vi "myRIO_BRig_FPGA_v3,80__PortC.vi"() -> ()   [LabVIEW 2014]
uses:
  <vilib>/rvi/Emulation/niFpgaGetClockAttributes.vi
  <vilib>/rvi/Emulation/niFpgaSctlEmulationGetInTimedLoop.vi
  <vilib>/rvi/Emulation/niFpgaEmulationReportErrorSimple.vi
  <vilib>/rvi/eio/common/nirviEmuTemplateMethod_errors.vi
  <vilib>/rvi/Emulation/niFpgaCriticalErrorInLSC.vi
  <vilib>/eio/EIONode/EIONode.xnode
panel:
  in  "I_allReward":bool
  in  "AnaOut_1":i16
  in  "CueLed_Event":bool
  in  "CueLed_nValley":u32=100
  in  "CueLed_nPeak":u32=100
  in  "LC_Event_l2":bool
  in  "LC_Laser_l2":bool
  in  "LC_nShutter_l2":u32=100
  in  "LC_nValley_l2":u32=100
  in  "LC_nPeak_l2":u32=100
  in  "LR_wrong_nDelay_l2":u32
  in  "LR_reward_nDelay_l2":u32
  in  "LR_wrong_nTotal_l2":u32=100
  in  "LR_reward_nTotal_l2":u32=100
  in  "LR_wrong_laser_l2":bool
  in  "LR_wrong_Event_l2":bool
  in  "LR_reward_Laser_l2":bool
  in  "LR_reward_Event_l2":bool
  out "AnaIn_1":i16
  out "AnaIn_0":i16
  out "timeTrial_count":u32
  in  "timeTrial_trig":bool
  in  "k1__counter_per_ms":u16=100 min=100 max=40000 step=1
  in  "LC_nShutter_l1":u32=100
  in  "AnaOut_0":i16
  in  "LC_nValley_l1":u32=100
  in  "LC_nPeak_l1":u32=100
  in  "LC_Event_l1":bool
  in  "LR_wrong_nTotal_l1":u32=100
  in  "LR_wrong_nDelay_l1":u32
  in  "LR_reward_nTotal_l1":u32=100
  in  "LR_reward_nDelay_l1":u32
  in  "LR_reward_Event_l1":bool
  in  "LR_wrong_Event_l1":bool
  out "SelectWrong":bool
  out "SelectReward":bool
  in  "LR_wrong_Laser_l1":bool
  in  "LR_reward_Laser_l1":bool
  in  "Left(F)_or_Right(T)":bool
  in  "ignoreWrong":bool
  in  "SelectionState":bool
  in  "LC_Laser_l1":bool
  in  "FPGA_Stop":bool
  in  "audioTrigger_L":bool
  in  "audioTrigger_R":bool
  in  "audioFreq_L_kHz":u8=14 min=1 max=14 step=1
  in  "audioAmp_L":u16=1 min=1 max=32767 step=1
  in  "audioFreq_R_kHz":u8=14 min=1 max=14 step=1
  in  "audioAmp_R":u16=1 min=1 max=32767 step=1
  in  "A3_SL":bool
  in  "A1_SR":bool
  in  "Counts_Reset":bool
  out "A4_LickR":u32
  out "A2_LickL":u32
  in  "A6_Act":bool
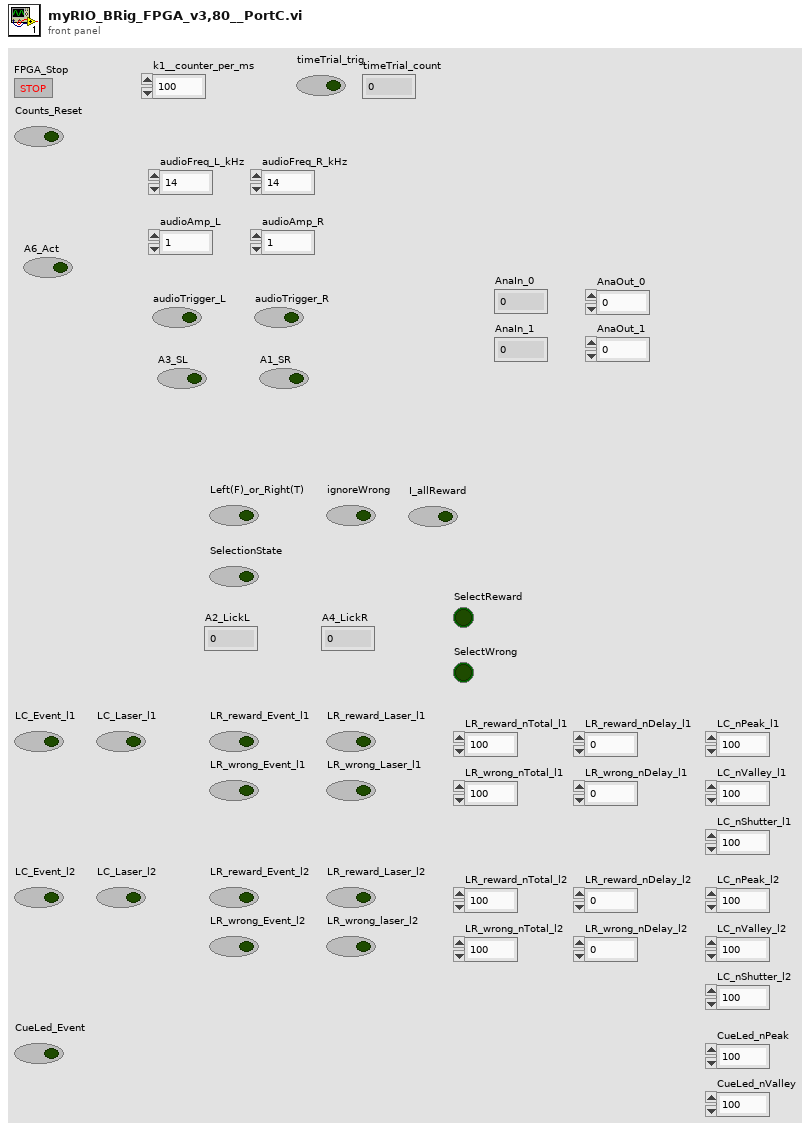
[diagram p1: front panel]
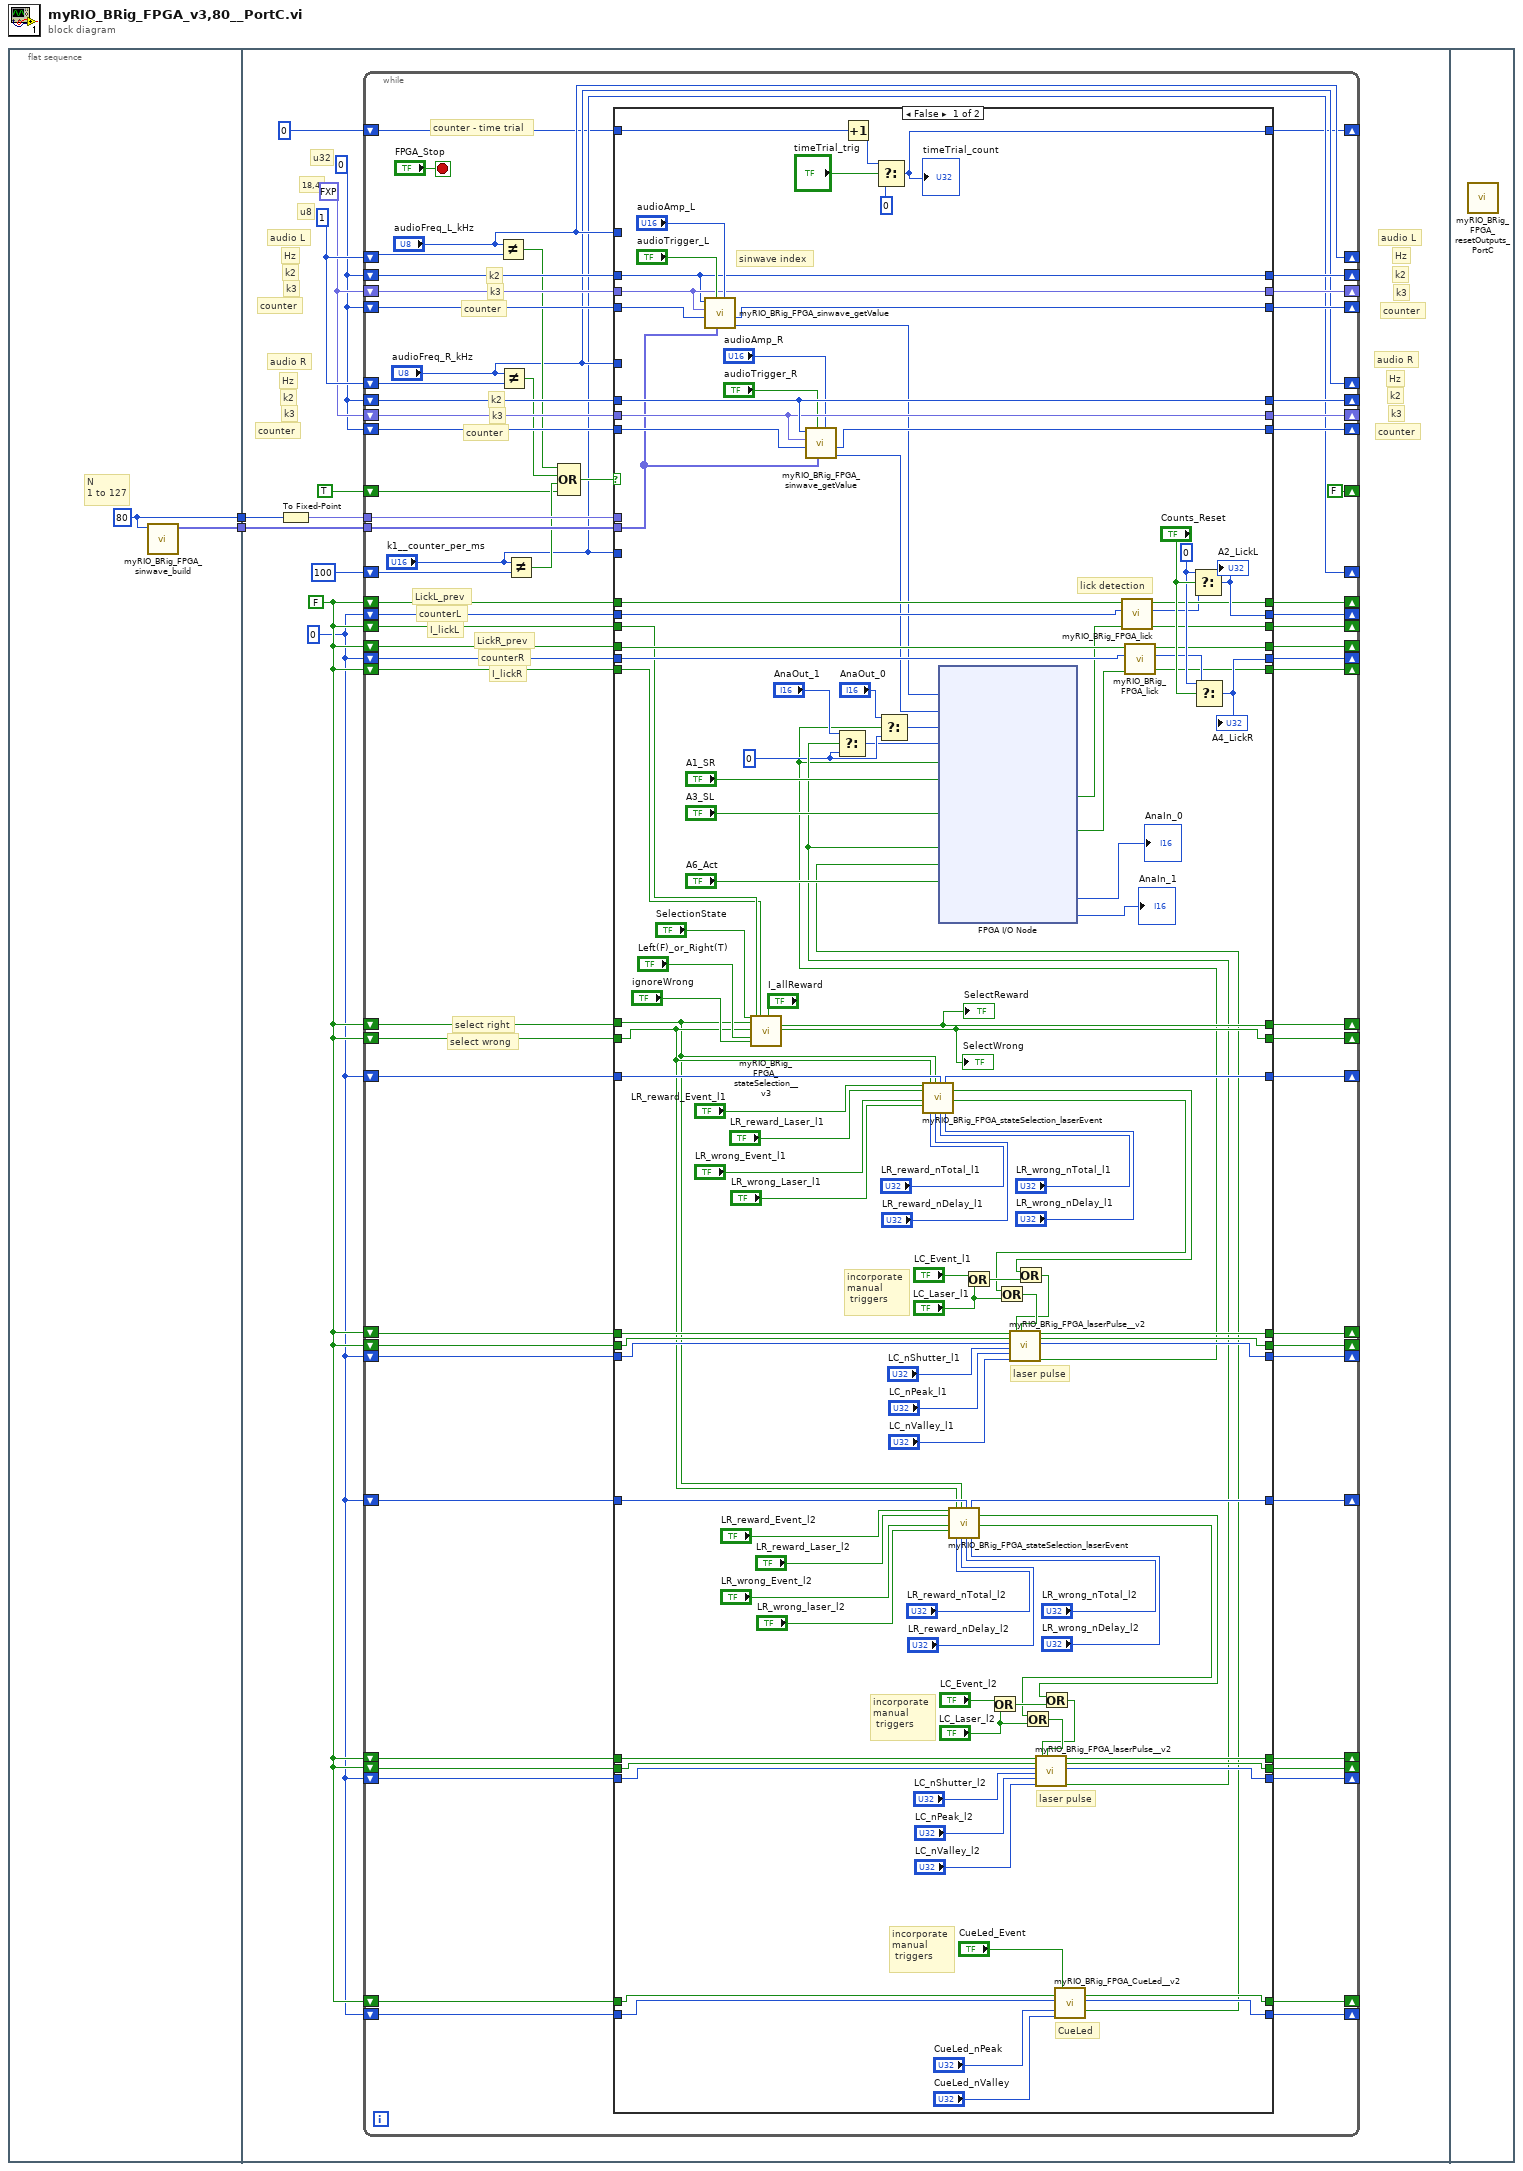
[diagram p0: block diagram]
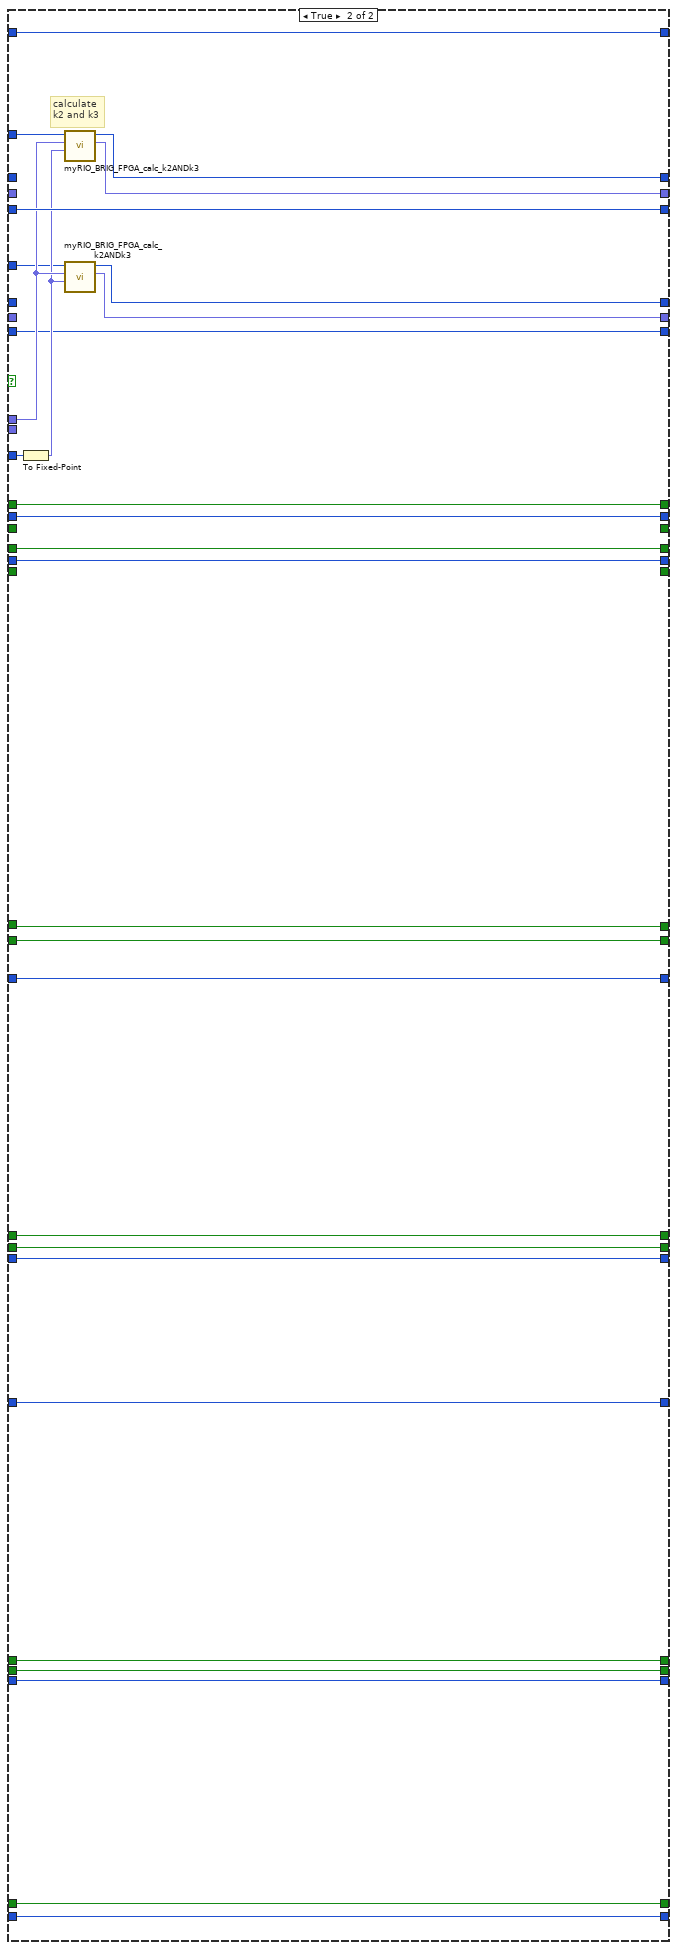
[diagram p2: hidden frame]
diagram:
  n1 = flat-sequence {
    tunnel: [w4] -> w2
    tunnel: [w3] -> w1
    tunnel: w2 -> [w15]
    tunnel: w1 -> [w14]
    frame #0 {
      w3 = 80 ("dimension size")
      # "N\n1 to 127"
      n2 = call "myRIO_BRig_FPGA_sinwave_build.vi"("input_Npts"=w3) -> ("output_array_sin"=w4:fxp<+/-,16,2>[])  [unwired: 10 in]
    }
    frame #1 {
      w5 = u32 0
      w6 = FALSE
      w10 = u32 0
      w11 = fxp<+,18,4> 0.0
      w12 = u8 1
      # "counter"
      # "k3"
      # "k2"
      # "counter"
      # "k3"
      # "k2"
      # "counter"
      # "counter"
      # "u32"
      # "k3"
      # "k2"
      # "k3"
      # "18,4"
      # "u8"
      # "Hz"
      # "Hz"
      # "audio R"
      # "audio L"
      # "Hz"
      # "k2"
      # "Hz"
      # "audio R"
      # "audio L"
      n3 = To Fixed-Point(number=w14) -> (fixed-point=w13:fxp<+,7,7>)  [unwired: 1 in]
      n4 = while {
        shift-right: ["audioFreq_L_kHz"] -> _
        shift-left: w12 -> [w80]
        shift-right: [w74] -> _
        shift-left: w10 -> [w78]
        shift-right: ["audioFreq_R_kHz"] -> _
        shift-left: w12 -> [w70]
        tunnel: w15 -> [w77]
        tunnel: w13 -> [w76]
        shift-right: [w73] -> _
        shift-left: w11 -> [w75]
        shift-right: [w71] -> _
        shift-left: w10 -> [w72]
        shift-right: [w68] -> _
        shift-left: w10 -> [w69]
        shift-right: [w66] -> _
        shift-left: w11 -> [w67]
        shift-right: [w64] -> _
        shift-left: w10 -> [w65]
        shift-right: ["k1__counter_per_ms"] -> _
        shift-left: u16 100 ("y") -> [w63]
        shift-right: [FALSE] -> _
        shift-left: TRUE -> [w58]
        shift-right: [w51] -> _
        shift-left: w6 -> [w53]
        shift-right: [w50] -> _
        shift-left: w6 -> [w52]
        shift-right: [w48] -> _
        shift-left: w5 -> [w49]
        shift-right: [w46] -> _
        shift-left: w5 -> [w47]
        shift-right: [w43] -> _
        shift-left: w6 -> [w45]
        shift-right: [w42] -> _
        shift-left: w6 -> [w44]
        shift-right: [w40] -> _
        shift-left: w6 -> [w41]
        shift-right: [w38] -> _
        shift-left: w6 -> [w39]
        shift-right: [w36] -> _
        shift-left: u32 0 -> [w37]
        shift-right: [w34] -> _
        shift-left: w5 -> [w35]
        shift-right: [w33] -> _
        shift-left: w6 -> [w30]
        shift-right: [w32] -> _
        shift-left: w6 -> [w29]
        shift-right: [w31] -> _
        shift-left: w5 -> [w28]
        shift-right: [w26] -> _
        shift-left: w5 -> [w27]
        shift-right: [w25] -> _
        shift-left: w6 -> [w22]
        shift-right: [w24] -> _
        shift-left: w6 -> [w21]
        shift-right: [w23] -> _
        shift-left: w5 -> [w20]
        shift-right: [w19] -> _
        shift-left: w6 -> [w17]
        shift-right: [w18] -> _
        shift-left: w5 -> [w16]
        stop <- "FPGA_Stop" stop-if-true
        # "counter"
        # "k3"
        # "k2"
        # "counter"
        # "k3"
        # "k2"
        # "counter - time trial"
        # "I_lickR"
        # "counterR"
        # "LickR_prev"
        # "I_lickL"
        # "counterL"
        # "LickL_prev"
        # "select wrong"
        # "select right"
        n5 = Not Equal?(x="audioFreq_L_kHz", y=w80) -> (x != y?=w62:bool)
        n6 = Not Equal?(x="audioFreq_R_kHz", y=w70) -> (x != y?=w61:bool)
        n7 = Not Equal?(x="k1__counter_per_ms", y=w63) -> (x != y?=w59:bool)
        n8 = Compound Arithmetic op=OR(w62, w61, w59, w58) -> (w60:bool)
        n9 = case shown="False" w60 {
          tunnel: w78 -> [w183 _]
          tunnel: "audioFreq_L_kHz" -> [_ w225]
          tunnel: w77 -> [w176 _]
          tunnel: w76 -> [_ w221]
          tunnel: "k1__counter_per_ms" -> [_ w226]
          tunnel: w75 -> [w184 _]
          tunnel: [w183 w224] -> w74
          tunnel: [w184 w223] -> w73
          tunnel: w72 -> [w188 w222]
          tunnel: [w185 w222] -> w71
          tunnel: w69 -> [w180 _]
          tunnel: [w180 w217] -> w68
          tunnel: w67 -> [w179 _]
          tunnel: [w179 w218] -> w66
          tunnel: w65 -> [w182 w216]
          tunnel: "audioFreq_R_kHz" -> [_ w219]
          tunnel: [w181 w216] -> w64
          tunnel: w53 -> [w171 w215]
          tunnel: w52 -> [w170 w214]
          tunnel: [w175 w215] -> w51
          tunnel: [w168 w214] -> w50
          tunnel: w49 -> [w172 w213]
          tunnel: [w198 w213] -> w48
          tunnel: w47 -> [w169 w212]
          tunnel: [w195 w212] -> w46
          tunnel: w45 -> [w103 w211]
          tunnel: w44 -> [w104 w210]
          tunnel: [w140 w211] -> w43
          tunnel: [w191 w210] -> w42
          tunnel: [w161 w207] -> w33
          tunnel: [w162 w206] -> w32
          tunnel: [w163 w205] -> w31
          tunnel: w41 -> [w165 _]
          tunnel: [w174 _] -> w40
          tunnel: w39 -> [w164 _]
          tunnel: [w166 _] -> w38
          tunnel: w37 -> [w153 w209]
          tunnel: [w150 w209] -> w36
          tunnel: w35 -> [w139 w208]
          tunnel: [w138 w208] -> w34
          tunnel: w30 -> [w129 w207]
          tunnel: w29 -> [w128 w206]
          tunnel: w28 -> [w127 w205]
          tunnel: w27 -> [w108 w204]
          tunnel: [w107 w204] -> w26
          tunnel: [w101 w203] -> w25
          tunnel: [w100 w202] -> w24
          tunnel: [w99 w201] -> w23
          tunnel: w22 -> [w98 w203]
          tunnel: w21 -> [w97 w202]
          tunnel: w20 -> [w96 w201]
          tunnel: [w93 w200] -> w19
          tunnel: [w92 w199] -> w18
          tunnel: w17 -> [w91 w200]
          tunnel: w16 -> [w90 w199]
          frame False {
            w85 = i16 0 ("f")
            w196 = u32 0 ("t")
            # "CueLed"
            # "incorporate\nmanual\n triggers"
            # "laser pulse"
            # "incorporate\nmanual\n triggers"
            # "sinwave index"
            # "lick detection"
            # "laser pulse"
            # "incorporate\nmanual\n triggers"
            n10 = call "myRIO_BRig_FPGA_sinwave_getValue.vi"("audioAmp"="audioAmp_L", "sinwave"=w176, "audioTrigger"="audioTrigger_L", "counter"=w188, "k3"=w184, "k2"=w183) -> ("output_audioValue"=w148:i16, "output_counter"=w185:u32)  [unwired: 4 in]
            n11 = call "myRIO_BRig_FPGA_stateSelection__v3.vi"("I_selectionState"="SelectionState", "I_selectRight"=w103, "I_selectWrong"=w104, "I_Left(F)_or_Right(T)"="Left(F)_or_Right(T)", "I_ignoreWrong"="ignoreWrong", "I_lickL"=w165, "I_lickR"=w164, "I_allReward"="I_allReward") -> ("output__I_selectRight"=w140:bool, "output__I_selectWrong"=w191:bool)  [unwired: 18 in]
            "SelectWrong" <- w191
            "SelectReward" <- w140
            n12 = call "myRIO_BRig_FPGA_sinwave_getValue.vi"("audioAmp"="audioAmp_R", "sinwave"=w176, "audioTrigger"="audioTrigger_R", "counter"=w182, "k3"=w179, "k2"=w180) -> ("output_audioValue"=w147:i16, "output_counter"=w181:u32)  [unwired: 4 in]
            n13 = Increment(x=w153) -> (x+1=w152:u32)
            n14 = Select(t=w152, s="timeTrial_trig", f=u32 0) -> (s? t:f=w150:u32)
            "timeTrial_count" <- w150
            n15 = call "myRIO_BRig_FPGA_stateSelection_laserEvent.vi"("I_LR_reward"="LR_reward_Event_l1", "I_LR_reward_laser"="LR_reward_Laser_l1", "I_LR_wrong"="LR_wrong_Event_l1", "I_LR_wrong_laser"="LR_wrong_Laser_l1", "I_selectWrong"=w104, "laser_reward_nTotal"="LR_reward_nTotal_l1", "I_selectReward"=w103, "laser_reward_nDelay"="LR_reward_nDelay_l1", "counter"=w139, "laser_wrong_nTotal"="LR_wrong_nTotal_l1", "laser_wrong_nDelay"="LR_wrong_nDelay_l1") -> ("output_counter"=w138:u32, "output_I_laserEvent"=w126:bool, "output_I_laserOn"=w125:bool)  [unwired: 6 in]
            n16 = call "myRIO_BRig_FPGA_stateSelection_laserEvent.vi"("I_LR_reward"="LR_reward_Event_l2", "I_LR_reward_laser"="LR_reward_Laser_l2", "I_LR_wrong"="LR_wrong_Event_l2", "I_LR_wrong_laser"="LR_wrong_laser_l2", "I_selectWrong"=w104, "laser_reward_nTotal"="LR_reward_nTotal_l2", "I_selectReward"=w103, "laser_reward_nDelay"="LR_reward_nDelay_l2", "counter"=w108, "laser_wrong_nTotal"="LR_wrong_nTotal_l2", "laser_wrong_nDelay"="LR_wrong_nDelay_l2") -> ("output_counter"=w107:u32, "output_I_laserEvent"=w102:bool, "output_I_laserOn"=w109:bool)  [unwired: 6 in]
            n17 = Or(x="LC_Event_l1", y="LC_Laser_l1") -> (x .or. y?=w157:bool)
            n18 = Or(x="LC_Event_l2", y="LC_Laser_l2") -> (x .or. y?=w119:bool)
            n19 = Or(x=w125, y="LC_Laser_l1") -> (x .or. y?=w155:bool)
            n20 = Or(x=w126, y=w157) -> (x .or. y?=w154:bool)
            n21 = call "myRIO_BRig_FPGA_laserPulse__v2.vi"("I_shutter"=w129, "I_peak"=w128, "count"=w127, "laser_Nshutter"="LC_nShutter_l1", "laser_Npeak"="LC_nPeak_l1", "laser_Nvalley"="LC_nValley_l1", "I_laserEvent"=w154, "I_laser"=w155) -> ("output_I_shutter"=w161:bool, "output_I_peak"=w162:bool, "output_count"=w163:u32, "output_laser"=w83:bool)  [unwired: 6 in, 2 out]
            n22 = Select(t="AnaOut_0", s=w83, f=w85) -> (s? t:f=w87:i16)
            n23 = Or(x=w109, y="LC_Laser_l2") -> (x .or. y?=w117:bool)
            n24 = Or(x=w102, y=w119) -> (x .or. y?=w116:bool)
            n25 = call "myRIO_BRig_FPGA_laserPulse__v2.vi"("I_shutter"=w98, "I_peak"=w97, "count"=w96, "laser_Nshutter"="LC_nShutter_l2", "laser_Npeak"="LC_nPeak_l2", "laser_Nvalley"="LC_nValley_l2", "I_laserEvent"=w116, "I_laser"=w117) -> ("output_I_shutter"=w101:bool, "output_I_peak"=w100:bool, "output_count"=w99:u32, "output_laser"=w86:bool)  [unwired: 6 in, 2 out]
            n26 = Select(t="AnaOut_1", s=w86, f=w85) -> (s? t:f=w82:i16)
            n27 = call "myRIO_BRig_FPGA_CueLed__v2.vi"("I_peak"=w91, "count"=w90, "laser_Npeak"="CueLed_nPeak", "laser_Nvalley"="CueLed_nValley", "I_CueLed_Event"="CueLed_Event") -> ("output_I_peak"=w93:bool, "output_count"=w92:u32, "output_led"=w89:bool)  [unwired: 12 in]
            n28 = xnode "FPGA I/O Node"("AudioOut/Left"=w148, "AudioOut/Right"=w147, "ConnectorC/AO0"=w87, "ConnectorC/AO1"=w82, "ConnectorC/DIO0"=w83, "ConnectorC/DIO1"="A1_SR", "ConnectorC/DIO3"="A3_SL", "ConnectorC/DIO5"=w86, "ConnectorC/DIO6"=w89, "ConnectorC/DIO7"="A6_Act") -> ("ConnectorC/DIO2"=w146:bool, "ConnectorC/DIO4"=w145:bool, "ConnectorC/AI0"=→"AnaIn_0":i16, "ConnectorC/AI1"=→"AnaIn_1":i16)  [unwired: 14 in, 14 out]
            n29 = call "myRIO_BRig_FPGA_lick.vi"("I_stateDetector_new"=w146, "counter"=w172, "I_stateDetector_prev"=w171) -> ("output_I_lick"=w174:bool, "output_counter"=w173:u32, "output_I_stateDetector_prev"=w175:bool)  [unwired: 6 in]
            n30 = call "myRIO_BRig_FPGA_lick.vi"("I_stateDetector_new"=w145, "counter"=w169, "I_stateDetector_prev"=w170) -> ("output_I_lick"=w166:bool, "output_counter"=w167:u32, "output_I_stateDetector_prev"=w168:bool)  [unwired: 6 in]
            n31 = Select(t=w196, s="Counts_Reset", f=w173) -> (s? t:f=w198:u32)
            "A2_LickL" <- w198
            n32 = Select(t=w196, s="Counts_Reset", f=w167) -> (s? t:f=w195:u32)
            "A4_LickR" <- w195
          }
          frame True {
            # "calculate\nk2 and k3"
            n33 = To Fixed-Point(number=w226) -> (fixed-point=w220:fxp<+,16,16>)  [unwired: 1 in]
            n34 = call "myRIO_BRIG_FPGA_calc_k2ANDk3.vi"("input_k1[count/ms]"=w220, "input_Npts"=w221, "input_freq[kHz]"=w225) -> ("output_k3"=w223:fxp<+,18,4>, "output_k2"=w224:u32)  [unwired: 7 in]
            n35 = call "myRIO_BRIG_FPGA_calc_k2ANDk3.vi"("input_k1[count/ms]"=w220, "input_Npts"=w221, "input_freq[kHz]"=w219) -> ("output_k3"=w218:fxp<+,18,4>, "output_k2"=w217:u32)  [unwired: 7 in]
          }
        }
      }
    }
    frame #2 {
      n36 = call "myRIO_BRig_FPGA_resetOutputs_PortC.vi"() -> ()  [unwired: 12 in]
    }
  }
